vi "PickUpTotes.vi"(8 "RC?":bool, 11 "Boolean Out":bool) -> (3 "Boolean":bool)   [LabVIEW 2014]
uses:
  Support Files/RC PickupStates.ctl
  Support Files/Global Data!!!.vi
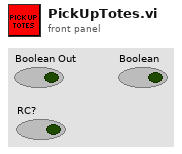
[diagram p1: front panel]
types:
  T1 = typedef "RC PickupStates.ctl" = enum16{"PickToteUp", "Disengage", "Drop", "Hold", "Lift", "Engage1Stage", "Rest", "DropAgain", "Done", "Lift.5", "Pause4Jones"}
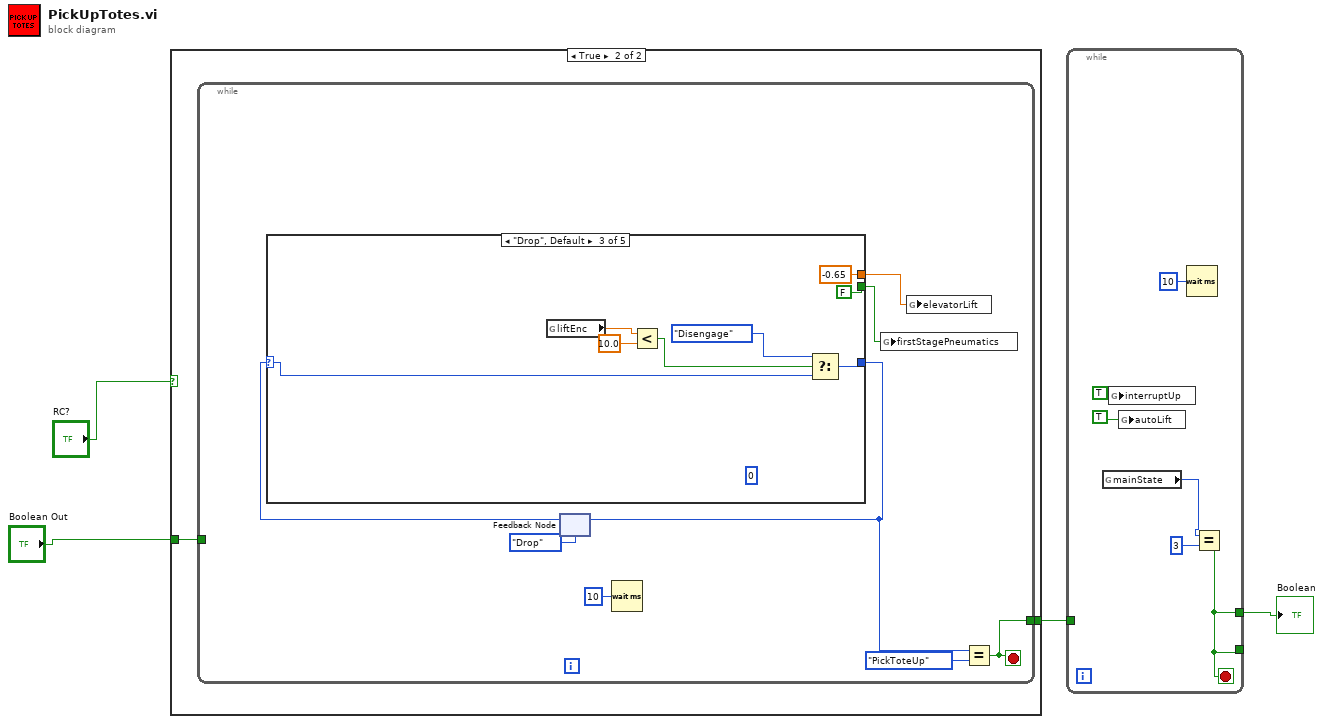
[diagram p0: block diagram]
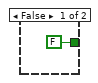
[diagram p2: hidden frame]
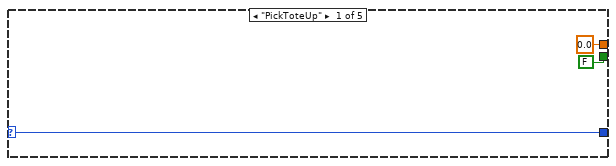
[diagram p3: hidden frame]
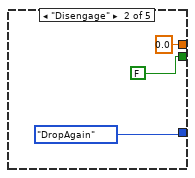
[diagram p4: hidden frame]
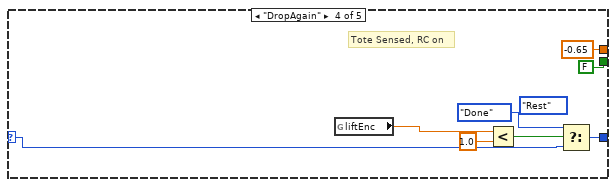
[diagram p5: hidden frame]
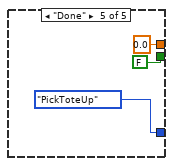
[diagram p6: hidden frame]
diagram:
  n1 = case shown="True" "RC?" {
    tunnel: "Boolean Out" -> [_ w7]
    tunnel: [FALSE w6] -> w2
    frame False {
    }
    frame True {
      n2 = while {
        tunnel: w7 -> [_]
        tunnel: [w8] -> w6
        stop <- w8 stop-if-true
        n3 = feedback #1(RC_PickupStates."Drop" ("t")) -> (w14:T1)
        n4 = case shown="\"Drop\", Default" w14 {
          selector: w14 -> [w18 _ w28 w36 _]
          tunnel: [FALSE FALSE FALSE ("Stage1?") FALSE ("Stage1?") FALSE ("Stage1?")] -> w12
          tunnel: [w18 RC_PickupStates."DropAgain" w29 w37 RC_PickupStates."PickToteUp"] -> w10
          tunnel: [0.0 0.0 -0.65 -0.65 0.0] -> w11
          frame "PickToteUp" {
          }
          frame "Disengage" {
          }
          frame "Drop", Default {
            (unwired) 0 ("t")
            n5 = global read "Global Data!!!.vi" "liftEnc"() -> (w26:dbl)
            n6 = Less?(x=w26, y=10.0) -> (x < y?=w24:bool)
            n7 = Select(t=RC_PickupStates."Disengage", s=w24, f=w28) -> (s? t:f=w29:T1)
          }
          frame "DropAgain" {
            (unwired) RC_PickupStates."Rest"
            # "Tote Sensed, RC on"
            n8 = global read "Global Data!!!.vi" "liftEnc"() -> (w33:dbl)
            n9 = Less?(x=w33, y=1.0) -> (x < y?=w34:bool)
            n10 = Select(t=RC_PickupStates."Done", s=w34, f=w36) -> (s? t:f=w37:T1)
          }
          frame "Done" {
          }
        }
        n11 = feedback-in #1(w10) -> ()
        n12 = Wait (ms)(milliseconds to wait=u32 10) -> ()  [unwired: 1 out]
        n13 = global write "Global Data!!!.vi" "firstStagePneumatics"(w12) -> ()
        n14 = global write "Global Data!!!.vi" "elevatorLift"(w11) -> ()
        n15 = Equal?(x=w10, y=RC_PickupStates."PickToteUp") -> (x = y?=w8:bool)
      }
    }
  }
  n16 = while {
    tunnel: w2 -> [_]
    tunnel: [w43] -> _
    tunnel: [w43] -> w1
    stop <- w43 stop-if-true
    n17 = global read "Global Data!!!.vi" "mainState"() -> (w45:i8)
    n18 = global write "Global Data!!!.vi" "interruptUp"(TRUE ("autoLift")) -> ()
    n19 = global write "Global Data!!!.vi" "autoLift"(TRUE ("autoLift")) -> ()
    n20 = Wait (ms)(milliseconds to wait=u32 10) -> ()  [unwired: 1 out]
    n21 = Equal?(x=w45, y=i8 3) -> (x = y?=w43:bool)
  }
  "Boolean" <- w1
